vi "Child UIDs.vi"(11 "Base Actor in":refnum<class "Base Actor.lvclass">) -> (2 "Child UIDs":T1)   [LabVIEW 2025, in "jettl.lvlib" / "Actor.lvlib" / "Base Actor.lvclass"]
uses:
  Base Actor.lvclass
  Base Actor.lvclass/Base Actor.ctl
  Child UIDs.ctl
  Actor.lvlib
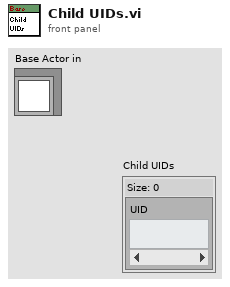
[diagram p1: front panel]
types:
  T1 = typedef "jettl.lvlib/Actor.lvlib/Child UIDs.ctl" = set{string}
  T2 = typedef "jettl.lvlib/Actor.lvlib/Base Actor.lvclass/Child Attributes Map.ctl" = map{string, refnum<class "Attributes.lvclass">}
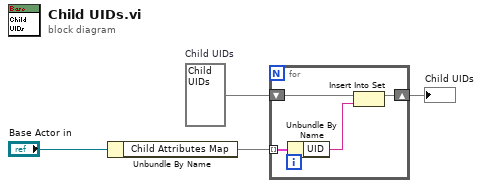
[diagram p0: block diagram]
diagram:
  w3 = T1 {}  # Child UIDs
  n1 = Unbundle By Name("Base Actor in") -> ("Child Attributes Map"=w1:T2)
  n2 = for {
    shift-right: [w7] -> w2
    shift-left: w3 -> [w8]
    tunnel: w1 -> [w5] mode=indexing
    n3 = Unbundle By Name(w5) -> ("UID"=w6:string)
    n4 = Insert Into Set(10:w6, 11:w8) -> (3:w7:T1)  [unwired: 1 out]
  }
  "Child UIDs" <- w2
